vi "CSV_import_control_lasers_and_SMs_and_ICC4C_importing_THORCAM.vi"() -> ()   [LabVIEW 2021]
uses:
  <vilib>/DAQmx/write.llb/DAQmx Write (Analog 1D DBL NChan 1Samp).vi
  <vilib>/Utility/file.llb/Read Delimited Spreadsheet (DBL).vi
  <vilib>/DAQmx/create/channels.llb/DAQmx Create Channel (AO-Voltage-Basic).vi
  C:/Program Files/Thorlabs/Scientific Imaging/DCx Camera Support/Develop/DotNet/uc480DotNet.dll
  Program Files/Thorlabs/Scientific Imaging/DCx Camera Support/Develop/DotNet/uc480DotNet.dll
panel:
  out "Full Cycles 2":i32
  in  "Interset Delay":i32
  in  "Interstep Delay":i32
  in  "ICC4C 3 (0-10V)":dbl
  in  "ICC4C 2 (0-10V)":dbl
  in  "ICC4C 1 (0-10V)":dbl
  in  "ICC4C 0 (0-10V)":dbl
  in  "Y2 (-10-10V)":dbl
  in  "X2 (-10-10V)":dbl
  in  "Continue Cycle?":bool
  out "Full Cycles":i32
  out "Phase I Iterations":i32
  out "Y1 (-10-10V)":dbl format="%_6g"
  out "X1 (-10-10V)":dbl format="%_6g"
  in  "Blanking (0-10v)":dbl=10.0
  in  "561 (0-10v)":dbl
  in  "514 (0-10v)":dbl
  in  "488 (0-10v)":dbl
  in  "445 (0-10v)":dbl
  # "NOTE: This starts at 0,  and will be end up  1 lower than the expected number of steps."
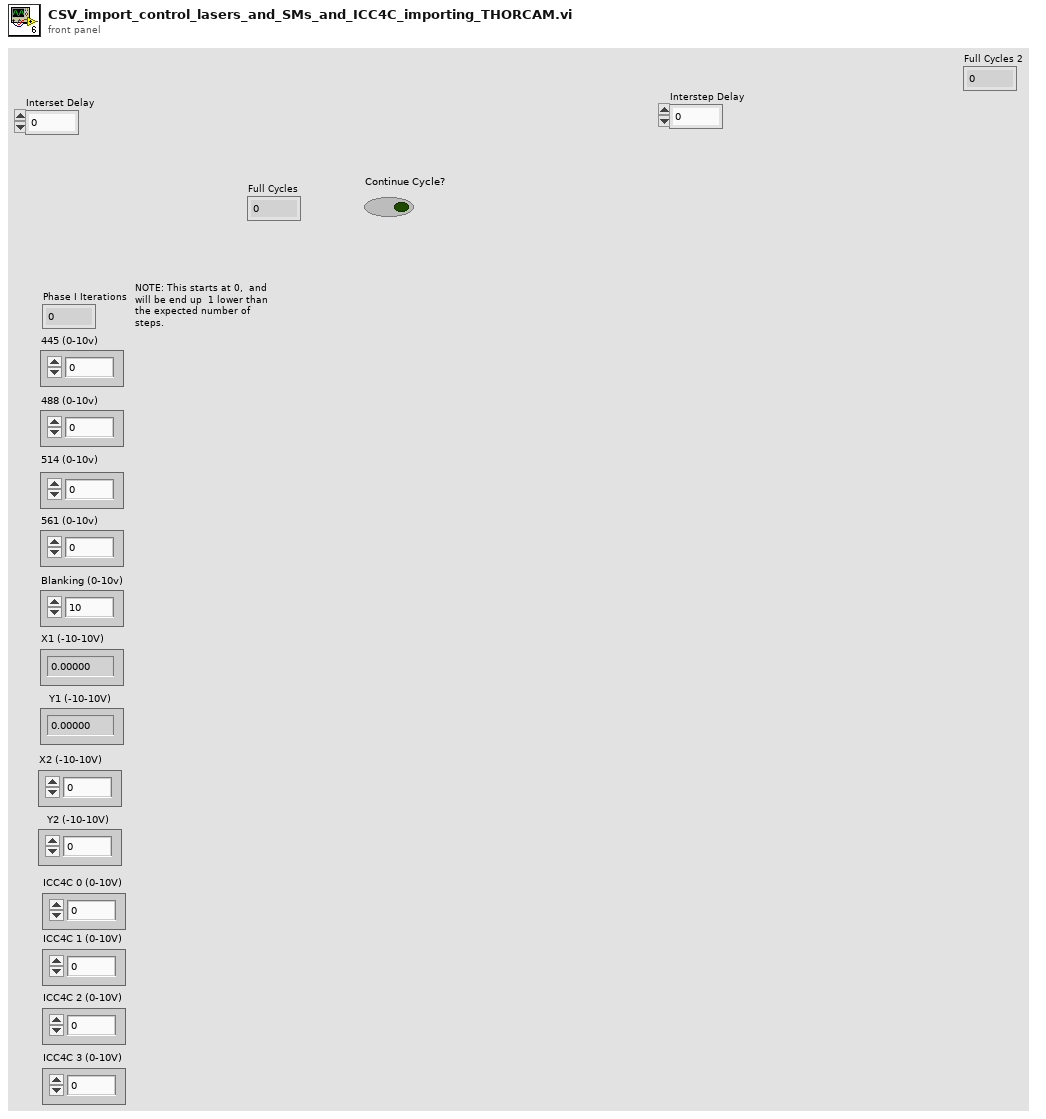
[diagram p1: front panel]
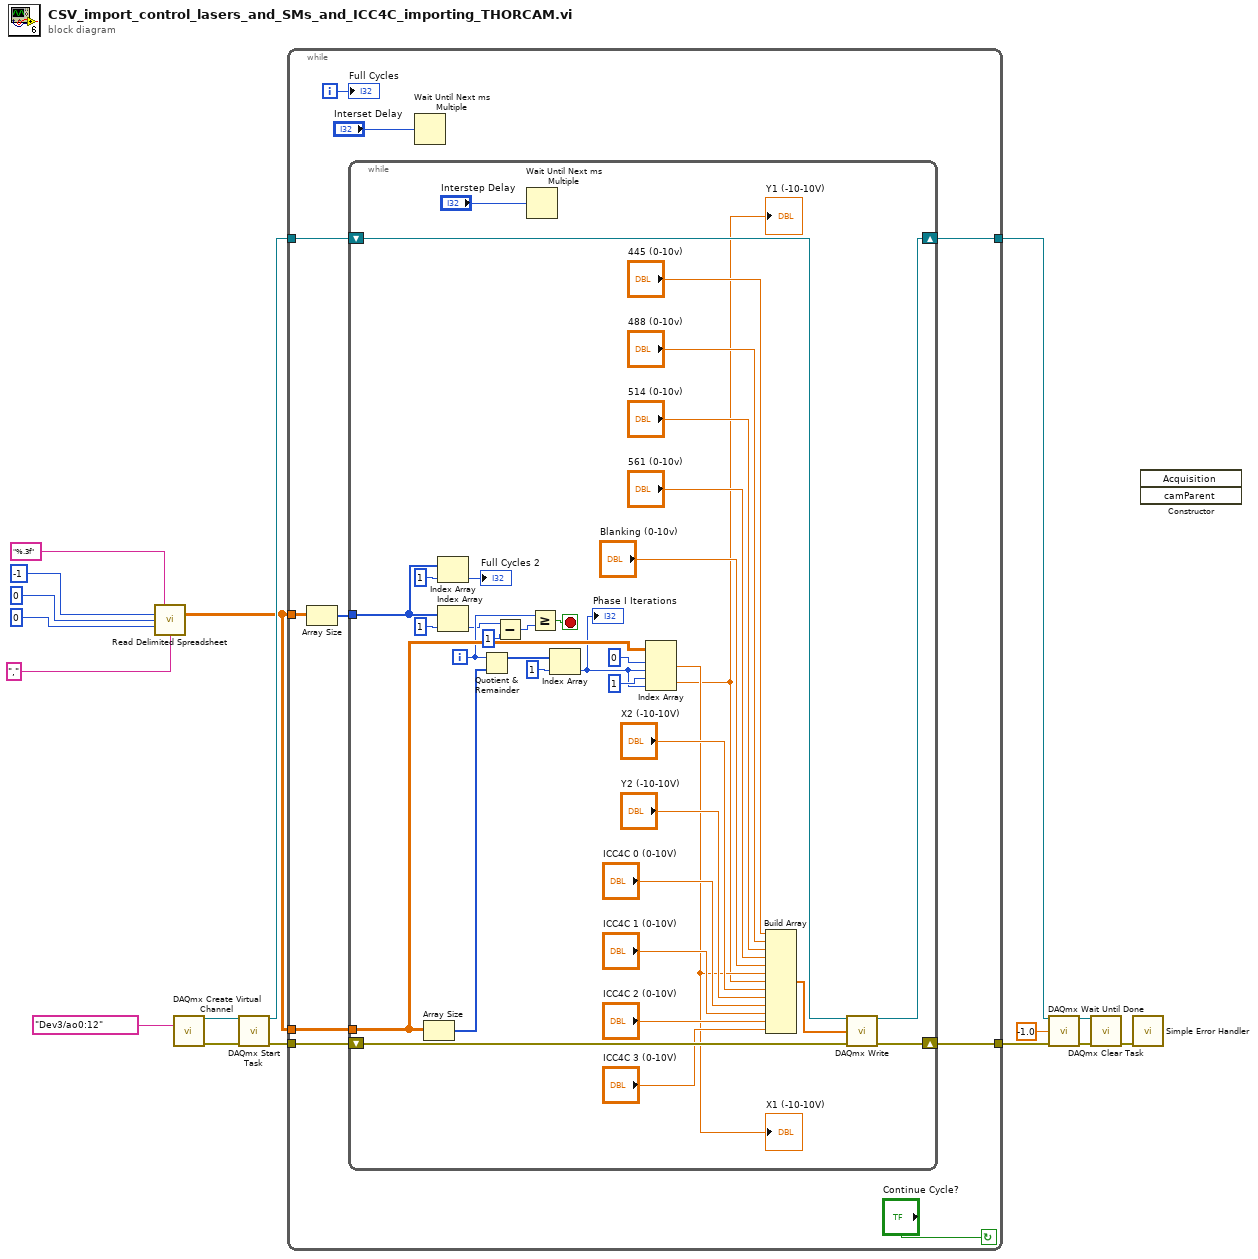
[diagram p0: block diagram]
diagram:
  n1 = call-poly <vilib>:"Read Delimited Spreadsheet.vi"("format (%.3f)"="%.3f", "number of rows (all:-1)"=-1, "start of read offset (chars.:0)"=0, "max characters/row  (no limit:0)"=0, "delimiter (\\t)"=",") -> ("all rows"=w6:dbl[][])  [unwired: 5 in, 5 out]
  n2 = call-poly <vilib>:"DAQmx Create Virtual Channel.vi"("physical channels"=tag "Dev3/ao0:12") -> ("task out"=w10:refnum<k21>, "error out"=w9:errorcluster)  [unwired: 13 in]
  n3 = call <vilib>:"DAQmx Start Task.vi"("task/channels in"=w10, "error in"=w9) -> ("task out"=w8:refnum<k21>, "error out"=w7:errorcluster)  [unwired: 12 in]
  n4 = while {
    tunnel: [w23] -> w13
    tunnel: [w22] -> w12
    tunnel: w8 -> [w26]
    tunnel: w7 -> [w25]
    tunnel: w6 -> [w20]
    tunnel: w6 -> [w19]
    i -> [w27]
    stop <- "Continue Cycle?" continue-if-true
    n5 = Array Size(array=w20) -> (size(s)=w21:i32[])
    n6 = while {
      shift-right: [w60] -> w23
      shift-left: w26 -> [w62]
      shift-right: [w59] -> w22
      shift-left: w25 -> [w61]
      tunnel: w21 -> [w33]
      tunnel: w19 -> [w41]
      i -> [w39]
      stop <- w31 stop-if-true
      n7 = Array Size(array=w41) -> (size(s)=w40:i32[])
      n8 = Index Array(array=w33, index=1) -> (element=→"Full Cycles 2":i32)
      n9 = Index Array(array=w33, index=1) -> (element=w30:i32)
      n10 = Quotient & Remainder(x=w39, y=w40) -> (x-y*floor(x/y)=w38:i32[])  [unwired: 1 out]
      n11 = Subtract(x=w30, y=1) -> (x-y=w29:i32)
      n12 = Wait Until Next ms Multiple(millisecond multiple="Interstep Delay") -> ()  [unwired: 1 out]
      n13 = Greater Or Equal?(x=w39, y=w29) -> (x >= y?=w31:bool)
      n14 = Index Array(array=w38, index=1) -> (element=w34:i32)
      "Phase I Iterations" <- w34
      n15 = Index Array(array=w41, index (row) #1=0, index (col) #1=w34, index (row) #2=1, index (col) #2=w34) -> (element #1=w45:dbl, element #2=w44:dbl)
      "X1 (-10-10V)" <- w45
      "Y1 (-10-10V)" <- w44
      n16 = Build Array("445 (0-10v)", "488 (0-10v)", "514 (0-10v)", "561 (0-10v)", "Blanking (0-10v)", w45, w44, "X2 (-10-10V)", "Y2 (-10-10V)", "ICC4C 0 (0-10V)", "ICC4C 1 (0-10V)", "ICC4C 2 (0-10V)", "ICC4C 3 (0-10V)") -> (w58:dbl[])
      n17 = call-poly <vilib>:"DAQmx Write.vi"("task/channels in"=w62, "data"=w58, "error in"=w61) -> ("task out"=w60:refnum<k21>, "error out"=w59:errorcluster)  [unwired: 10 in, 1 out]
    }
    n18 = Wait Until Next ms Multiple(millisecond multiple="Interset Delay") -> ()  [unwired: 1 out]
    "Full Cycles" <- w27
  }
  n19 = call <vilib>:"DAQmx Wait Until Done.vi"("task/channels in"=w13, "timeout (sec)"=-1.0, "error in"=w12) -> ("task out"=w16:refnum<k21>, "error out"=w15:errorcluster)  [unwired: 11 in]
  n20 = call <vilib>:"DAQmx Clear Task.vi"("task in"=w16, "error in"=w15) -> ("error out"=w17:errorcluster)  [unwired: 13 in]
  n21 = call <vilib>:"Simple Error Handler.vi"("error in (no error)"=w17) -> ()  [unwired: 4 in, 5 out]
  n22 = constructor class="Acquisition"() -> ()  [unwired: 4 in, 4 out]
